vi "PID Percentage to EGU.vi"   [LabVIEW 2017, in "NI_PID_pid.lvlib"]
doc: "Converts a percent-of-range input to an engineering-units output based on the minimum and maximum range settings. The output is normally limited to the range [max...min]. Values outside of the range [max..min] are allowed when <B>coerce output to range?</B> is FALSE. Use the DBL instance of this VI to implement a single control loop. Use the DBL Array instance to implement parallel multi-loop control."
uses:
  <vilib>/addons/control/pid/NI_PID_pid.lvlib
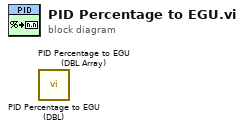
[diagram p0: block diagram]
diagram:
  n1 = call <vilib>:"PID Percentage to EGU (DBL).vi"() -> ()  [unwired: 4 in, 1 out]
  n2 = call <vilib>:"PID Percentage to EGU (DBL Array).vi"() -> ()  [unwired: 4 in, 1 out]
